vi "Replace Period with Underscore.vi"(1 "string":string) -> (0 "result string":string)   [LabVIEW 2020, in "Data.lvclass"]
uses:
  Data.lvclass
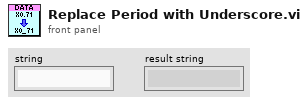
[diagram p1: front panel]
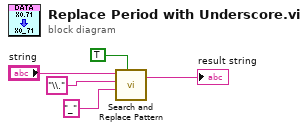
[diagram p0: block diagram]
diagram:
  n1 = call <vilib>:"Search and Replace Pattern.vi"("string"="string", "regular expression (\"\")"="\\." ("regular expression (\"\")"), "replace string (\"\")"="_" ("replace string (\"\")"), "replace all? (F)"=TRUE) -> ("result string"=→"result string":string)  [unwired: 1 in, 1 out]
